vi "Get Tx Generic Section and Channels.vi"(8 "error in":errorcluster, 11 "Custom Device Ref in":T1 format="%.0x") -> (0 "error out":errorcluster, 1 "Tx Queue Status channel Refs":T1[](array[typedef]) format="%.0x", 2 "Tx Queue Status Section Ref out":T1 format="%.0x", 3 "Custom Device Ref out":T1 format="%.0x", 4 "Found?":bool)   [LabVIEW 2020, in "AIM ARINC 664 Scripting.lvlib"]
uses:
  AIM ARINC 664 Scripting.lvlib
  <vilib>/NI VeriStand/Custom Device API/Custom Device Item Ref.ctl
  Constants.vi
  GUID Utility/AIM ARINC 664 GUID Utility.lvlib
  <vilib>/NI VeriStand/Custom Device API/Custom Device API.lvlib
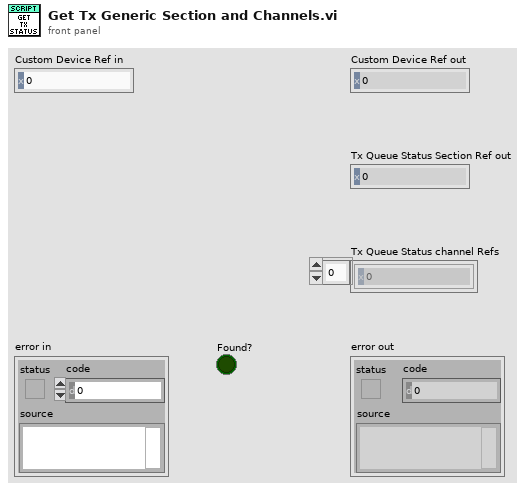
[diagram p1: front panel]
types:
  T1 = typedef "Custom Device API.lvlib/Custom Device Item Ref.ctl" = u64
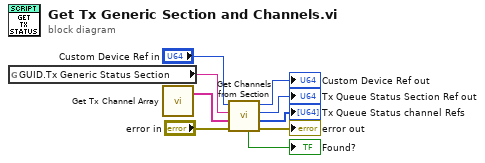
[diagram p0: block diagram]
diagram:
  n1 = global read "Constants.vi" "GUID.Tx Generic Status Section"() -> (w7:string)
  n2 = call "Get Tx Channel Array.vi"() -> ("Channel Array"=w2:string[])  [unwired: 3 in]
  n3 = call "Get Channels from Section.vi"("error in (no error)"="error in", "Channel Array"=w2, "GUID Section"=w7, "Custom Device Ref in"="Custom Device Ref in") -> ("error out"=→"error out":errorcluster, "Channel Array Refs"=→"Tx Queue Status channel Refs":T1[], "Section Ref"=→"Tx Queue Status Section Ref out":T1, "Custom Device Ref out"=→"Custom Device Ref out":T1, "All Channels Found"=→"Found?":bool)  [unwired: 3 in]
